vi "bandwidth adjustment.vi"() -> ()   [LabVIEW 2015]
uses:
  <vilib>/measure/NI_MAPro.lvlib
  <vilib>/measure/maspectr.llb/FFT Power Spectrum and PSD for N Chan.vi
  <vilib>/Waveform/DWDTOps.llb/DWDT Analog to Digital.vi
  <vilib>/Waveform/DWDTOps.llb/DWDT Digital to Binary U8.vi
  <vilib>/Waveform/DWDTOps.llb/DWDT Digital to Analog.vi
panel:
  in  "stop":bool
  out "Waveform Graph 2":i8[](graph)
  out "Array":bool[](array[boolean])
  out "8bit integer":i8[][](array[numeric])
  out "binary array":u32[](array[numeric])
  out "Digital Data 2":digitaldata={"transitions"=[], "data"=[[1, 1, 1, 1]]}
  out "Digital Waveform Graph":digitalwaveform(graph)
  out "full-scale range (out)":dbl
  out "resolution (out)":i32=16
  out "digital waveform 2":digitalwaveform(waveform)={"t0"=timestamp(0 s since 1904-01-01), "dt"=0.0, "Y"={"transitions"=[], "data"=[]}, "error"={"status"=FALSE, "code"=37421928, "source"=""}}
  in  "full-scale range (pk-pk)":dbl=2.0
  out "Time Domain":dynamicdata(graph)
  out "Frequency Domain":cluster{"f0":dbl, "df":dbl, "magnitude":dbl[]}[](graph)
  out "Waveform Graph":dynamicdata(graph)
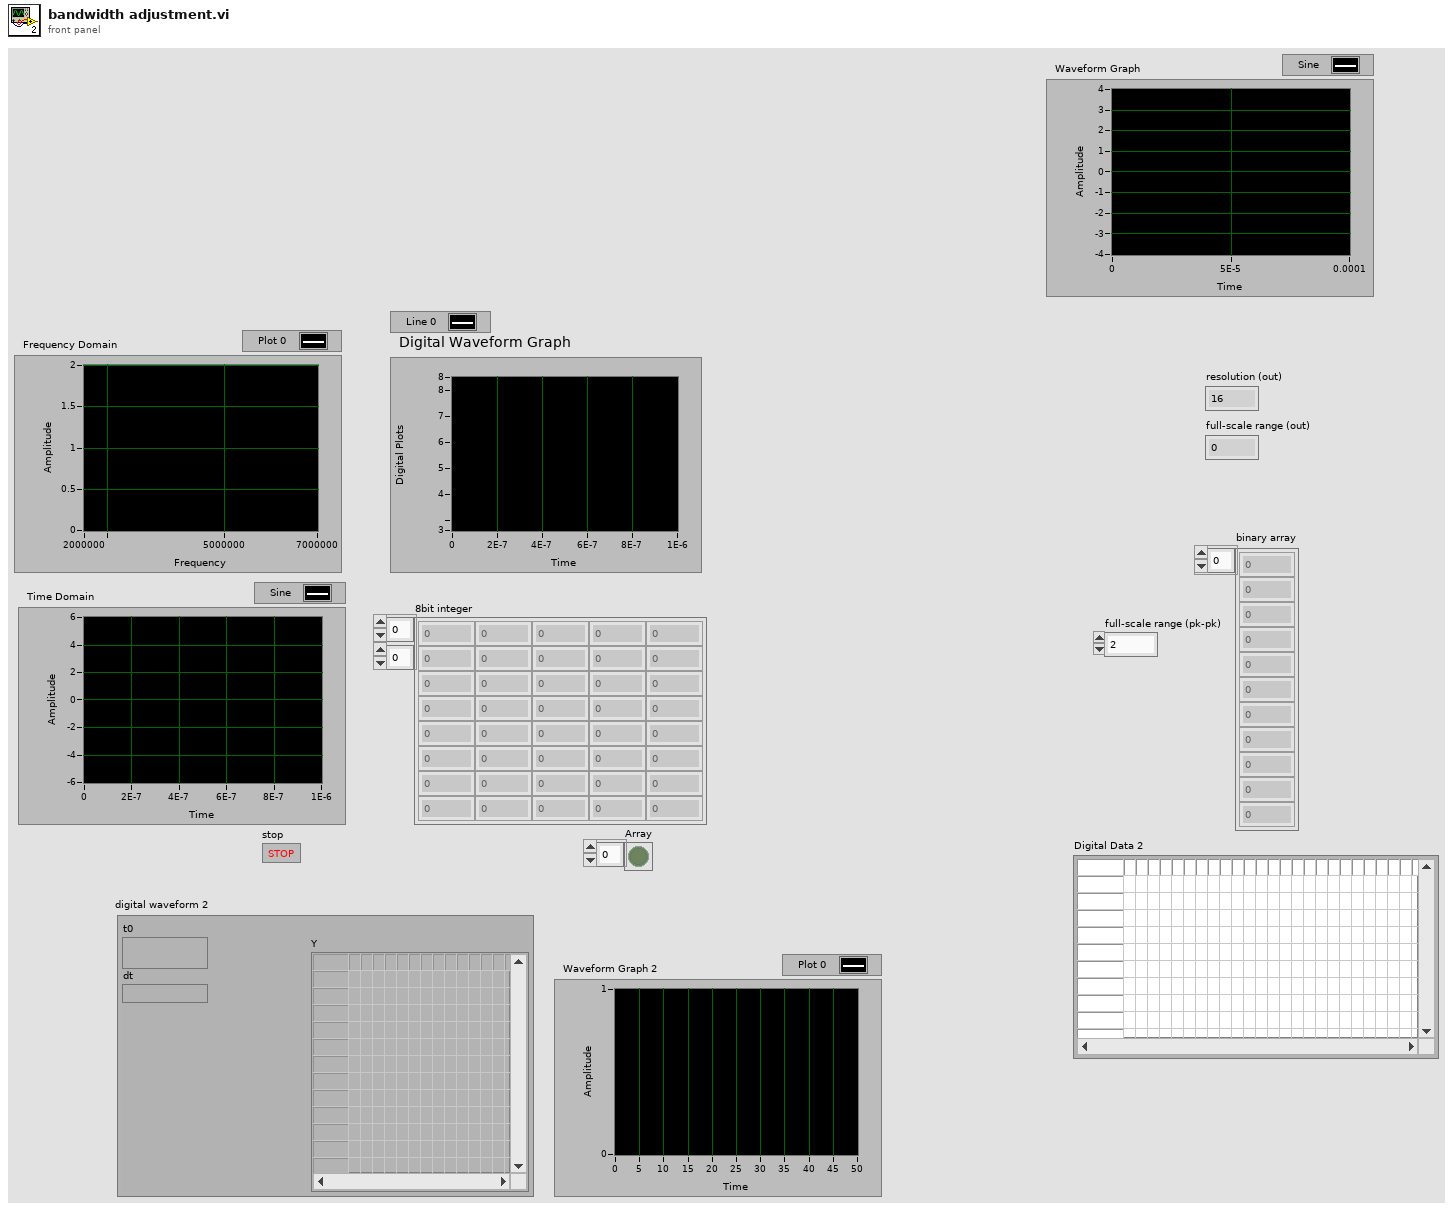
[diagram p1: front panel]
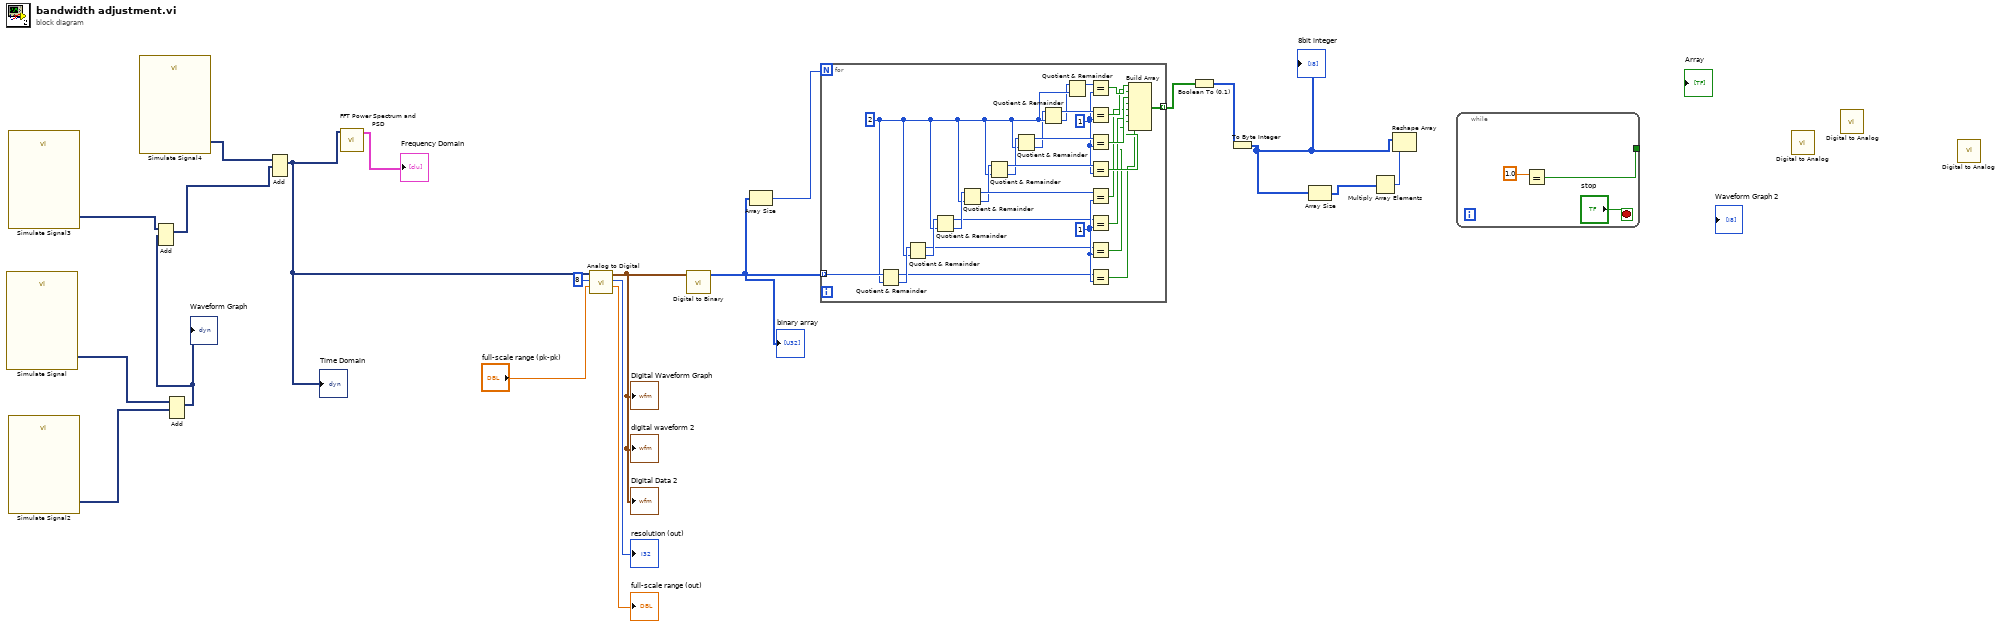
[diagram p0: block diagram]
diagram:
  n1 = call "Simulate Signal"() -> ("Sine"=w20:dynamicdata)  [unwired: 14 in, 1 out]
  n2 = call "Simulate Signal3"() -> ("Sine"=w18:dynamicdata)  [unwired: 14 in, 1 out]
  n3 = call "Simulate Signal2"() -> ("Sine"=w19:dynamicdata)  [unwired: 14 in, 1 out]
  n4 = call "Simulate Signal4"() -> ("Sine"=w16:dynamicdata)  [unwired: 14 in, 1 out]
  n5 = Add(1:w19, 2:w20) -> (0:w17:dynamicdata)  [unwired: 1 in, 1 out]
  "Waveform Graph" <- w17
  n6 = Add(1:w17, 2:w18) -> (0:w15:dynamicdata)  [unwired: 1 in, 1 out]
  n7 = Add(1:w15, 2:w16) -> (0:w2:dynamicdata)  [unwired: 1 in, 1 out]
  "Time Domain" <- w2
  n8 = call-poly <vilib>:"FFT Power Spectrum and PSD.vi"("time signals"=w2) -> ("Power Spectrum / PSD"=→"Frequency Domain":cluster{"f0":dbl, "df":dbl, "magnitude":dbl[]}[])  [unwired: 7 in, 3 out]
  n9 = call-poly <vilib>:"Analog to Digital.vi"("full-scale range (pk-pk)"="full-scale range (pk-pk)", "resolution (16 bit)"=8, "analog waveform"=w2) -> ("full-scale range (out)"=→"full-scale range (out)":dbl, "resolution (out)"=→"resolution (out)":i32, "digital waveform"=w10:digitalwaveform)  [unwired: 5 in, 1 out]
  "digital waveform 2" <- w10
  "Digital Waveform Graph" <- w10
  "Digital Data 2" <- w10
  n10 = call-poly <vilib>:"Digital to Binary.vi"("digital waveform"=w10) -> ("binary array"=w4:u8[])  [unwired: 9 in, 1 out]
  "binary array" <- w4
  n11 = Array Size(array=w4) -> (size(s)=w3:i32)
  n12 = for {
    N: w3 -> [_]
    tunnel: w4 -> [w44] mode=indexing
    tunnel: [w21] -> w8 mode=indexing
    w35 = 1
    w32 = 2
    w45 = 1
    n13 = Quotient & Remainder(x=w44, y=w32) -> (x-y*floor(x/y)=w43:i32, floor(x/y)=w46:i32)
    n14 = Quotient & Remainder(x=w46, y=w32) -> (x-y*floor(x/y)=w42:i32, floor(x/y)=w47:i32)
    n15 = Quotient & Remainder(x=w47, y=w32) -> (x-y*floor(x/y)=w41:i32, floor(x/y)=w48:i32)
    n16 = Quotient & Remainder(x=w48, y=w32) -> (x-y*floor(x/y)=w40:i32, floor(x/y)=w33:i32)
    n17 = Quotient & Remainder(x=w33, y=w32) -> (x-y*floor(x/y)=w36:i32, floor(x/y)=w34:i32)
    n18 = Quotient & Remainder(x=w34, y=w32) -> (x-y*floor(x/y)=w37:i32, floor(x/y)=w31:i32)
    n19 = Quotient & Remainder(x=w31, y=w32) -> (x-y*floor(x/y)=w38:i32, floor(x/y)=w30:i32)
    n20 = Quotient & Remainder(x=w30, y=w32) -> (x-y*floor(x/y)=w39:i32)  [unwired: 1 out]
    n21 = Equal?(x=w39, y=w35) -> (x = y?=w29:bool)
    n22 = Equal?(x=w38, y=w35) -> (x = y?=w28:bool)
    n23 = Equal?(x=w37, y=w35) -> (x = y?=w27:bool)
    n24 = Equal?(x=w36, y=w35) -> (x = y?=w26:bool)
    n25 = Equal?(x=w40, y=w45) -> (x = y?=w25:bool)
    n26 = Equal?(x=w41, y=w45) -> (x = y?=w24:bool)
    n27 = Equal?(x=w42, y=w45) -> (x = y?=w23:bool)
    n28 = Equal?(x=w43, y=w45) -> (x = y?=w22:bool)
    n29 = Build Array(w29, w28, w27, w26, w25, w24, w23, w22) -> (w21:bool[])
  }
  n30 = Boolean To (0,1)(Boolean=w8) -> (0, 1=w9:i16[][])
  n31 = To Byte Integer(number=w9) -> (8bit integer=w5:i8[][])
  "8bit integer" <- w5
  n32 = Array Size(array=w5) -> (size(s)=w7:i32[])
  n33 = Multiply Array Elements(1:w7) -> (0:w6:i32)
  n34 = Reshape Array(w5, w6) -> ()  [unwired: 1 out]
  n35 = while {
    tunnel: [w50] -> _
    stop <- "stop" stop-if-true
    n36 = Equal?(x=1.0) -> (x = y?=w50:bool)  [unwired: 1 in]
  }
  n37 = call-poly <vilib>:"Digital to Analog.vi"() -> ()  [unwired: 8 in, 4 out]
  n38 = call-poly <vilib>:"Digital to Analog.vi"() -> ()  [unwired: 8 in, 4 out]
  n39 = call-poly <vilib>:"Digital to Analog.vi"() -> ()  [unwired: 8 in, 4 out]
